vi "StrQueue-Set Event Case Timeout.vi"(2 "default":i32=-1, 7 "Quit":bool) -> (8 "timeout":i32)   [LabVIEW 2020]
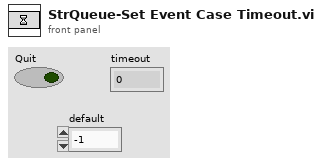
[diagram p1: front panel]
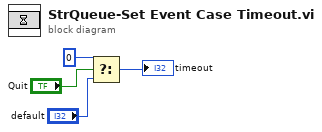
[diagram p0: block diagram]
diagram:
  n1 = Select(t=0, s="Quit", f="default") -> (s? t:f=→"timeout":i32)
